vi "Subset Digital Tach.vi"(5 "reset? (True)":bool=TRUE, 6 "Start":dbl format="%.2f", 7 "digital tach info":T1={"tacho counts"=[], "counter timebase [Hz]"=20000000.0, "counter task type"=enum."event counting", "counter digit (32)"=32}) -> (3 "digital tach info":T1={"tacho counts"=[], "counter timebase [Hz]"=20000000.0, "counter task type"=enum."event counting", "counter digit (32)"=32})   [LabVIEW 2017]
uses:
  <vilib>/addons/Sound and Vibration/Order Analysis/Tach Process/SubVIs/digital tach info.ctl
  <vilib>/addons/Sound and Vibration/Order Analysis/Tach Process/SoundVib_TachProcess.lvlib
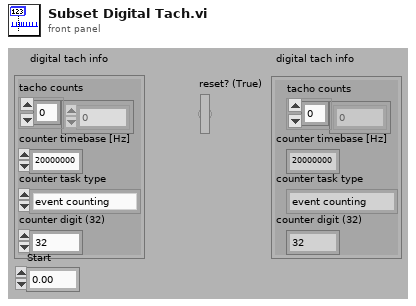
[diagram p1: front panel]
types:
  T1 = typedef "SoundVib_TachProcess.lvlib/digital tach info.ctl" = cluster{"tacho counts":i64[], "counter timebase [Hz]":dbl, "counter task type":enum16{"period measurement", "event counting"}, "counter digit (32)":i32}
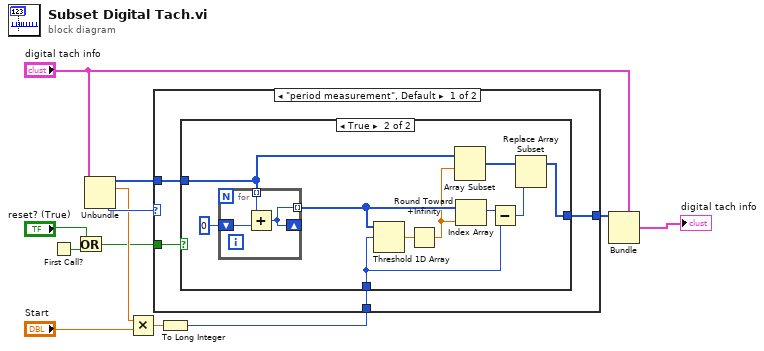
[diagram p0: block diagram]
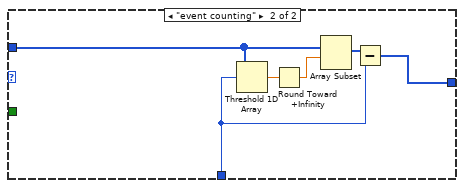
[diagram p3: hidden frame]
diagram:
  n1 = First Call?() -> (First Call?: T/F=w3:bool)
  n2 = Or(x="reset? (True)", y=w3) -> (x .or. y?=w1:bool)
  n3 = Unbundle("digital tach info") -> ("tacho counts"=w12:i64[], "counter timebase [Hz]"=w10:dbl, "counter task type"=w11:enum16{"period measurement", "event counting"})  [unwired: 1 out]
  n4 = Multiply(x=w10, y="Start") -> (x*y=w6:dbl)
  n5 = To Long Integer(number=w6) -> (32bit integer=w4:i32)
  n6 = case shown="\"period measurement\", Default" w11 {
    tunnel: w12 -> [w15 w32]
    tunnel: [w14 w31] -> w5
    tunnel: w4 -> [w16 w35]
    tunnel: w1 -> [w13 _]
    frame "period measurement", Default {
      n7 = case shown="True" w13 {
        tunnel: w16 -> [_ w25]
        tunnel: w15 -> [w17 w23]
        tunnel: [w17 w18] -> w14
        frame False {
        }
        frame True {
          n8 = for {
            shift-right: [w29] -> _
            shift-left: u32 0 -> [w30]
            tunnel: [w29] -> w27 mode=indexing
            tunnel: w23 -> [w28] mode=indexing
            n9 = Add(x=w28, y=w30) -> (x+y=w29:i64)
          }
          n10 = Threshold 1D Array(2:w25, 3:w27) -> (0:w26:dbl)  [unwired: 1 in]
          n11 = Round Toward +Infinity(x=w26) -> (ceil(x): smallest int >= x=w22:dbl)
          n12 = Array Subset(array=w23, index=w22) -> (w20:i64[])  [unwired: 1 in]
          n13 = Index Array(array=w27, index=w22) -> (element=w21:i64)
          n14 = Subtract(x=w21, y=w25) -> (x-y=w19:i64)
          n15 = Replace Array Subset(array=w20, new element=w19) -> (w18:i64[])  [unwired: 1 in]
        }
      }
    }
    frame "event counting" {
      n16 = Threshold 1D Array(2:w35, 3:w32) -> (0:w36:dbl)  [unwired: 1 in]
      n17 = Round Toward +Infinity(x=w36) -> (ceil(x): smallest int >= x=w34:dbl)
      n18 = Array Subset(array=w32, index=w34) -> (w33:i64[])  [unwired: 1 in]
      n19 = Subtract(x=w33, y=w35) -> (x-y=w31:i64[])
    }
  }
  n20 = Bundle(cluster="digital tach info", "tacho counts"=w5) -> (→"digital tach info":T1)  [unwired: 3 in]
